vi "Write Window Handle.vi"(8 "error in (no error)":errorcluster, 10 "Window Handle":i32, 11 "Measurement Setup UI in":refnum<class "Measurement Setup UI.lvclass">) -> (0 "error out":errorcluster, 3 "Measurement Setup UI out":refnum<class "Measurement Setup UI.lvclass">)   [LabVIEW 2016, in "Measurement Setup Controller.lvlib" / "Measurement Setup UI.lvclass"]
uses:
  Measurement Setup UI.lvclass
  Measurement Setup UI.lvclass/Measurement Setup UI.ctl
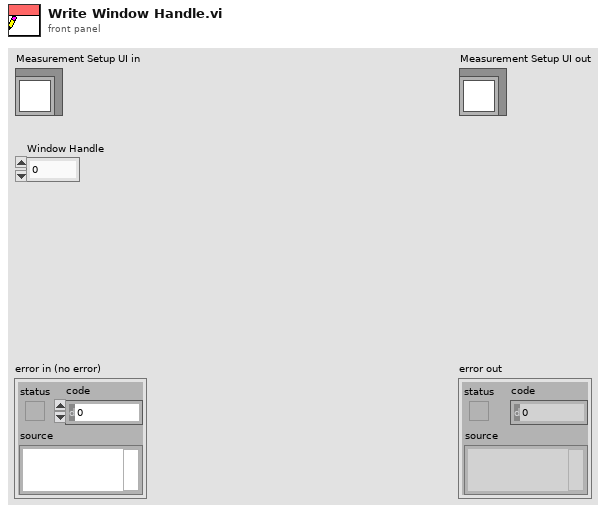
[diagram p1: front panel]
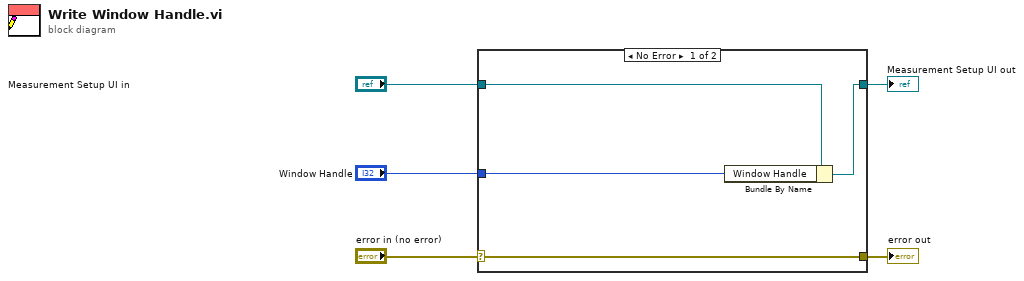
[diagram p0: block diagram]
diagram:
  n1 = case shown="No Error" "error in (no error)" {
    selector: "error in (no error)" -> [w9 w10]
    tunnel: [w9 w10] -> w4
    tunnel: [w7 w11] -> w2
    tunnel: "Measurement Setup UI in" -> [w8 w11]
    tunnel: "Window Handle" -> [w6 _]
    frame No Error {
      n2 = Bundle By Name(cluster=w8, "Window Handle"=w6) -> (w7:refnum<class "Measurement Setup UI.lvclass">)
    }
    frame Error {
    }
  }
  "error out" <- w4
  "Measurement Setup UI out" <- w2
